vi "Write String Properties.vi"(8 "error in (no error)":errorcluster, 10 "String Array Properties":T1[](array[typedef]), 11 "Item Ref in in":T2 format="%.0x") -> (0 "error out":errorcluster, 3 "Item Ref out":T2 format="%.0x")   [LabVIEW 2017, in "Engine Simulation Toolkit System Explorer.lvlib"]
uses:
  Engine Simulation Toolkit System Explorer.lvlib
  <vilib>/NI Veristand/Custom Device API/Custom Device Item Ref.ctl
  String Array Property.ctl
  <vilib>/NI Veristand/Custom Device API/Set Item Property (String Array).vi
  <vilib>/NI Veristand/Custom Device API/Custom Device API.lvlib
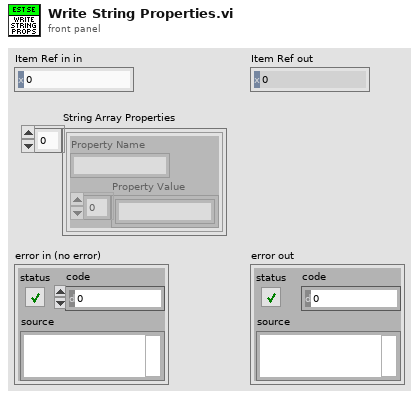
[diagram p1: front panel]
types:
  T1 = typedef "Engine Simulation Toolkit System Explorer.lvlib/String Array Property.ctl" = cluster{"Property Name":string, "Property Value":string[]}
  T2 = typedef "Custom Device API.lvlib/Custom Device Item Ref.ctl" = u64
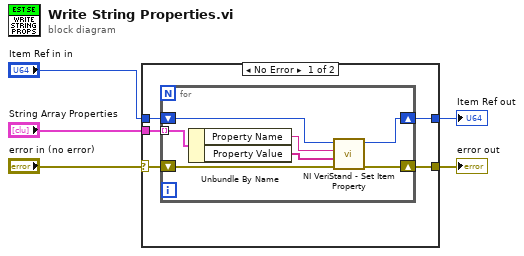
[diagram p0: block diagram]
diagram:
  n1 = case shown="No Error" "error in (no error)" {
    selector: "error in (no error)" -> [w7 w18]
    tunnel: [w10 w19] -> w5
    tunnel: "Item Ref in in" -> [w9 w19]
    tunnel: [w8 w18] -> w3
    tunnel: "String Array Properties" -> [w6 _]
    frame No Error {
      n2 = for {
        tunnel: w6 -> [w13] mode=indexing
        shift-right: [w16] -> w8
        shift-left: w7 -> [w17]
        shift-right: [w14] -> w10
        shift-left: w9 -> [w15]
        n3 = Unbundle By Name(w13) -> ("Property Name"=w12:string, "Property Value"=w11:string[])
        n4 = call-poly <vilib>:"NI VeriStand - Set Item Property.vi"("error in (no error)"=w17, "Value"=w11, "Property Name"=w12, "Item Ref in"=w15) -> ("error out"=w16:errorcluster, "Item Ref out"=w14:T2)  [unwired: 5 in, 1 out]
      }
    }
    frame Error {
    }
  }
  "Item Ref out" <- w5
  "error out" <- w3
